vi "LDA_Channel_Naming.vi"(2 "Numeric":i32, 3 "After May 2019":bool) -> (0 "Channel Name":string, 1 "No of Samples":string)   [LabVIEW 2018]
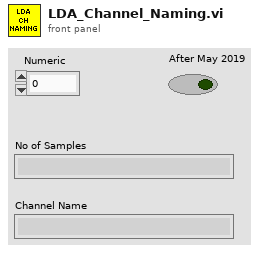
[diagram p1: front panel]
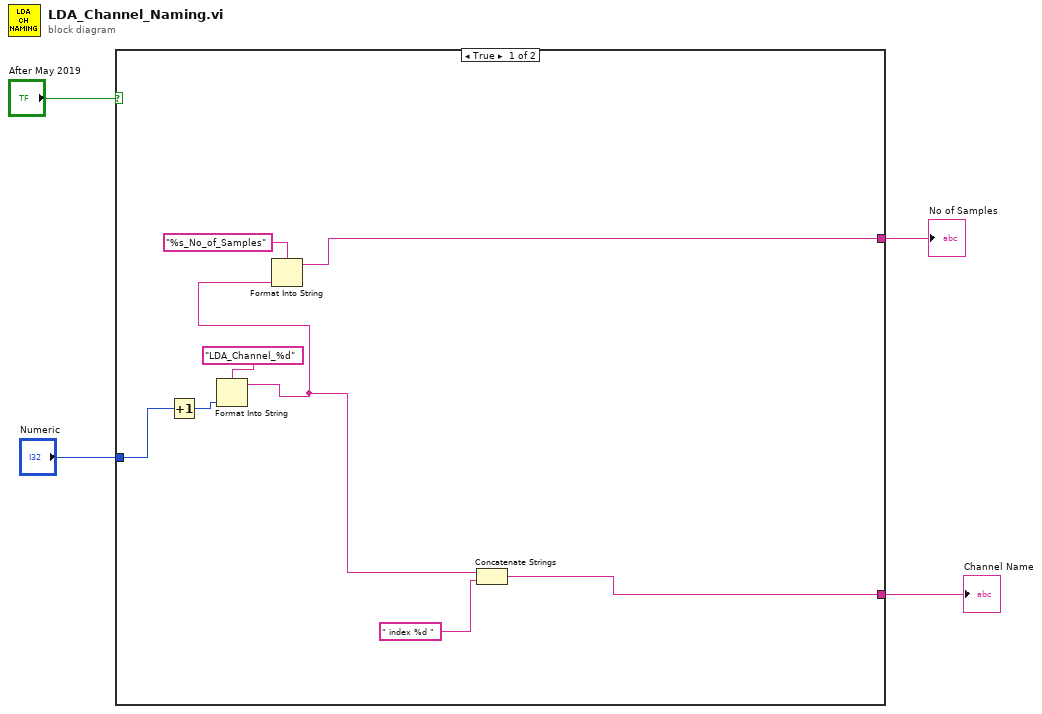
[diagram p0: block diagram]
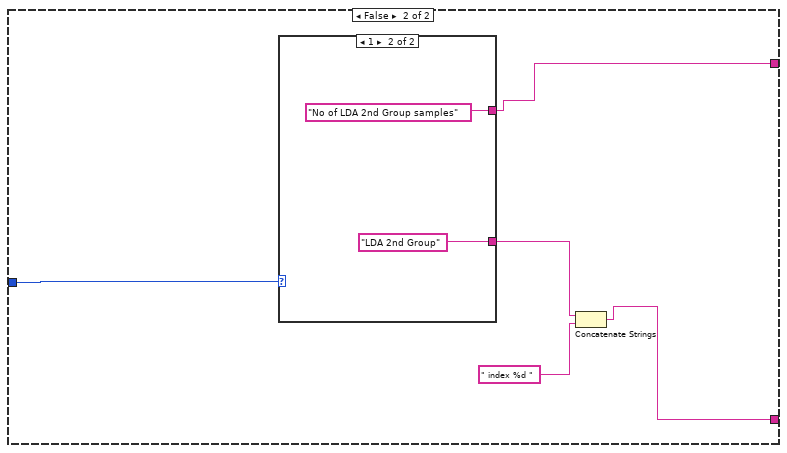
[diagram p2: hidden frame]
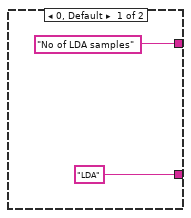
[diagram p3: hidden frame]
diagram:
  n1 = case shown="True" "After May 2019" {
    tunnel: "Numeric" -> [w9 w15]
    tunnel: [w8 w14] -> w3
    tunnel: [w5 w13] -> w2
    frame True {
      n2 = Increment(x=w9) -> (x+1=w10:i32)
      n3 = Format Into String(format string="LDA_Channel_%d", w10) -> (resulting string=w6:string)  [unwired: 2 in, 1 out]
      n4 = Format Into String(format string="%s_No_of_Samples", w6) -> (resulting string=w8:string)  [unwired: 2 in, 1 out]
      n5 = Concatenate Strings(w6, " index %d " ("format string")) -> (w5:string)
    }
    frame False {
      n6 = case shown="1" w15 {
        tunnel: ["LDA" ("format string") "LDA 2nd Group" ("format string")] -> w17
        tunnel: ["No of LDA samples" "No of LDA 2nd Group samples"] -> w14
        frame 0, Default {
        }
        frame 1 {
        }
      }
      n7 = Concatenate Strings(w17, " index %d " ("format string")) -> (w13:string)
    }
  }
  "Channel Name" <- w2
  "No of Samples" <- w3
